vi "IV.vi"(6 "Speed":enum16{"Normal", "Fast", "Instant"}(ring), 8 "error in":errorcluster, 11 "Transport":refnum<class "SMO.Transport.lvclass">) -> (0 "error out":errorcluster, 3 "Transport out":refnum<class "SMO.Transport.lvclass">)   [LabVIEW 2019, in "SMO.Transport.lvclass"]
uses:
  SMO.Transport.lvclass
  <userlib>/LevyLab/Lockin-Multichannel/Instrument.Lockin/Instrument.Lockin.lvclass
  SMO.Control Experiment/SMO.Control Experiment.lvclass
  <userlib>/LevyLab/Instrument Framework/Instrument Types/CBridge/Instrument.CBridge.lvclass
  <userlib>/LevyLab/Instrument Framework/Instrument Types/Cryostat/Instrument.Cryostat.lvclass
  <userlib>/LevyLab/Krohn Hite 7008/Instrument.KH7008.lvclass
  <userlib>/LevyLab/Instrument Framework/Instrument Types/Strain/Instrument.Strain.lvclass
  <userlib>/LevyLab/Instrument Framework/Instrument Types/VNA/Instrument.VNA.lvclass
  <userlib>/LevyLab/Instrument Framework/Instrument Types/VSource/Instrument.VSource.lvclass
  SMO.Control Experiment/Private/Control Experiment SM/Typedefs/Instruments--cluster.ctl
  <userlib>/LevyLab/Instrument Framework/Instrument Types/Delay Line/Instrument.DelayLine.lvclass
  <userlib>/LevyLab/Lockin-Multichannel/Instrument.DAQ/Typedefs/AO.Channel.Function--Enum.ctl
  <userlib>/LevyLab/Lockin-Multichannel/Instrument.DAQ/Instrument.DAQ.lvclass
  <userlib>/LevyLab/Lockin-Multichannel/Instrument.DAQ/Typedefs/AO.Channel--Cluster.ctl
  <userlib>/LevyLab/Lockin-Multichannel/Instrument.DAQ/Typedefs/AO.Channel--Cluster--Array.ctl
  <userlib>/_OpenG.lib/array/array.llb/Index 1D Array Elements (Variant)__ogtk.vi
panel:
  out "4Term":cluster{dbl[], dbl[]}[](graph)
  out "2Term":T1(graph)
  in  "Tab Control":T2(tab)
  in  "decimating factor":i32=5
  in  "low cutoff freq: fl":dbl=0.01 format="%0.4f"
  out "Temp (K)":dbl=0.013306618000000001
  in  "offset":dbl[](array[numeric])=[0.0, 0.0, 0.0, 0.0, 0.0, 0.0, 0.0, 0.0, 0.0, 0.0, 0.0, 0.0, 0.0, 0.0, 0.0, 0.0, 0.0, 0.0, 0.0, 0.0, 0.0, 0.0, 0.0, 0.0] format="%_6p"
  in  "invert":dbl[](array[numeric])=[1.0, 1.0, 1.0, 1.0, 1.0, 1.0, 1.0, 1.0, 1.0, 1.0, 1.0, 1.0, 1.0, 1.0, 1.0, 1.0, 1.0, 1.0, 1.0, 1.0, 1.0, 1.0, 1.0, 1.0] format="%#_6p"
  out "Field (T)":dbl=-0.0014
  in  "Enable Filter?":bool
  out "AI Waveform":waveform(dbl)[](graph)
  out "AO Waveform":waveform(dbl)[](graph)
  in  "AI indices":i32[](array[numeric])
  in  "AO indices":i32[](array[numeric])
  in  "Experiment Folder":string="test"
  in  "Experiment Comments":string="   IV measurements at 0T\n     - Sweep priority 0: +y gate from 25V to -25V in steps of 2V (-y -25 to 25)\n     - 1 IV curves at each Vsg\n     - KH channel 17,18,19,20: leads 3,8,15,27\n    Vbg = lead 26: 0V\n    T: 20mK\n    B=0T\n    \n    \n    400nm periodicity mesh\n    \n        KH channel 4,3: leads 7,6 , current mode, 5k resistor, 1000x gain\n        lead 7: 5mV ac+ 0uV dc bias, 0.02 Hz\n        KH channel 1,2: V1+/-: 4,5 1000x gain\n    \n    rectangle\n    \n        KH channel 7,6: leads 12,11, current mode, 5k resistor, 1000x gain\n        lead 12: 5mV ac+ 0uV dc bias, 0.02 Hz\n        KH channel 8,5: V1+/-: 13,9 1000x gain\n    \n    \n    200nm periodicity mesh\n    \n        KH channel 12,11: leads 16,17 , current mode, 5k resistor, 1000x gain\n        lead 21: 5mV ac+ 180uV dc bias, 0.02 Hz\n        KH channel 9,10: V1+/-: 21,20 1000x gain\n    \n    line filter on in lockin\n    decimating factor: 5"
  in  "OK":bool
  # "Speed:\n- Normal: The Lockin is \"paused\" and this program triggers an aquisition and waits for a new waveform. There is some program overhead so it takes slightly longer than acquisition time\n- Fast: Set the Lockin to be in running mode with whatever acquisition time you want (1 s, 2 s, 5 s, etc) and then this program acquires the waveforms and saves them. \n- Instant: There are NO checks to make sure that the waveform is different than the previous."
  # "*** These controls are only read if this VI is the top level. If is is called from Sweep Control then the folder and comments come from Sweep Control.vi ***"
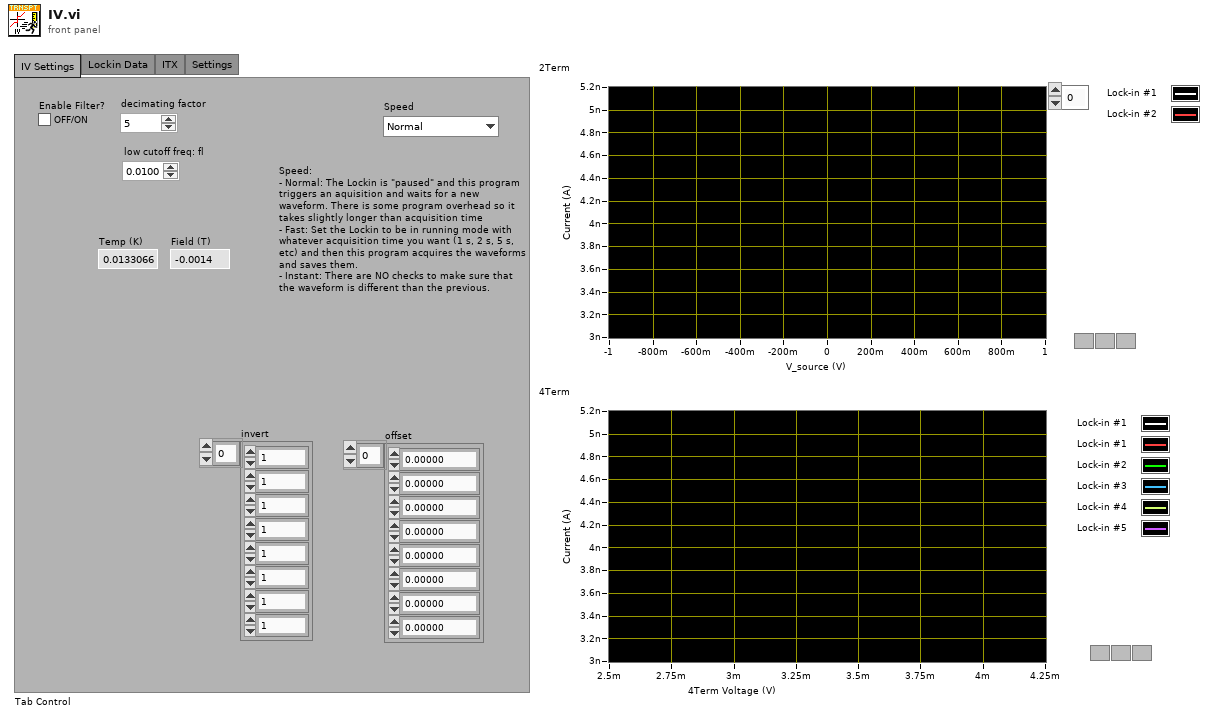
[diagram p1: front panel]
types:
  T1 = cluster{"Decimated and Filtered Array":dbl[], "Decimated and Filtered Array":dbl[]}[]
  T2 = enum32{"IV Settings", "Lockin Data", "ITX", "Settings"}
  T3 = enum32{"Invalid", "Standard", "Closed", "Hidden", "Minimized", "Maximized"}
  T4 = enum32{"invalid app kind", "Development System", "Run Time System", "Student Edition", "Embedded LabVIEW", "Evaluation", "Custom"}
  T5 = typedef "SMO.Control Experiment.lvclass/Instruments--cluster.ctl" = cluster{"Lockin":refnum<class "Instrument.Lockin.lvclass">, "Temperature":refnum<class "Instrument.Cryostat.lvclass">, "Magnet":refnum<class "Instrument.Cryostat.lvclass">, "Rotator":refnum<class "Instrument.Cryostat.lvclass">, "Level":refnum<class "Instrument.Cryostat.lvclass">, "C Bridge":refnum<class "Instrument.CBridge.lvclass">, "Optical Delay Line":refnum<class "Instrument.DelayLine.lvclass">, "Strain Cell":refnum<class "Instrument.Strain.lvclass">, "VNA":refnum<class "Instrument.VNA.lvclass">, "Voltage Source":refnum<class "Instrument.VSource.lvclass">, "KH7008":refnum<class "Instrument.KH7008.lvclass">[]}
  T6 = typedef "Instrument.DAQ.lvclass/AO.Channel--Cluster--Array.ctl" = T7[]
  T7 = typedef "Instrument.DAQ.lvclass/AO.Channel--Cluster.ctl" = cluster{"Enable?":bool, "Channel":i32, "Amplitude":dbl, "Offset":dbl, "Frequency":dbl, "Phase":dbl, "Function":T8, "Sweeping?":bool}
  T8 = typedef "Instrument.DAQ.lvclass/AO.Channel.Function--Enum.ctl" = enum16{"Sine", "Triangle", "Square"}
  T9 = cluster{"Core":cluster{"Current VI Reference":refnum<vi>, "Close Panel on Exit?":bool}, "Transport":refnum<class "SMO.Transport.lvclass">, "Control Experiment":refnum<class "SMO.Control Experiment.lvclass">, "Instruments":T5, "Temperature":dbl, "Magnet":dbl, "AOconfig":T6, "AO Waveforrm":waveform(dbl)[], "AI Waveform":waveform(dbl)[], "time":dbl[], "time (filtered)":dbl[], "AI (filtered)":cluster{"Decimated and Filtered Array":dbl[]}[], "AO (filtered)":cluster{"Decimated and Filtered Array":dbl[]}[], "Execution:State":enum32{"Bad", "Idle", "Run top level", "Running"}}
  T10 = enum32{"Bad", "Idle", "Run top level", "Running"}
  T11 = cluster{"Current VI Reference":refnum<vi>, "Close Panel on Exit?":bool}
  T12 = cluster{"I-":i32, "I+":i32, "V1-":i32, "V1+":i32, "I2-":i32, "I2+":i32, "V2-":i32, "V2+":i32}
  T13 = cluster{"Decimated and Filtered Array":dbl[], "Decimated and Filtered Array":dbl[]}
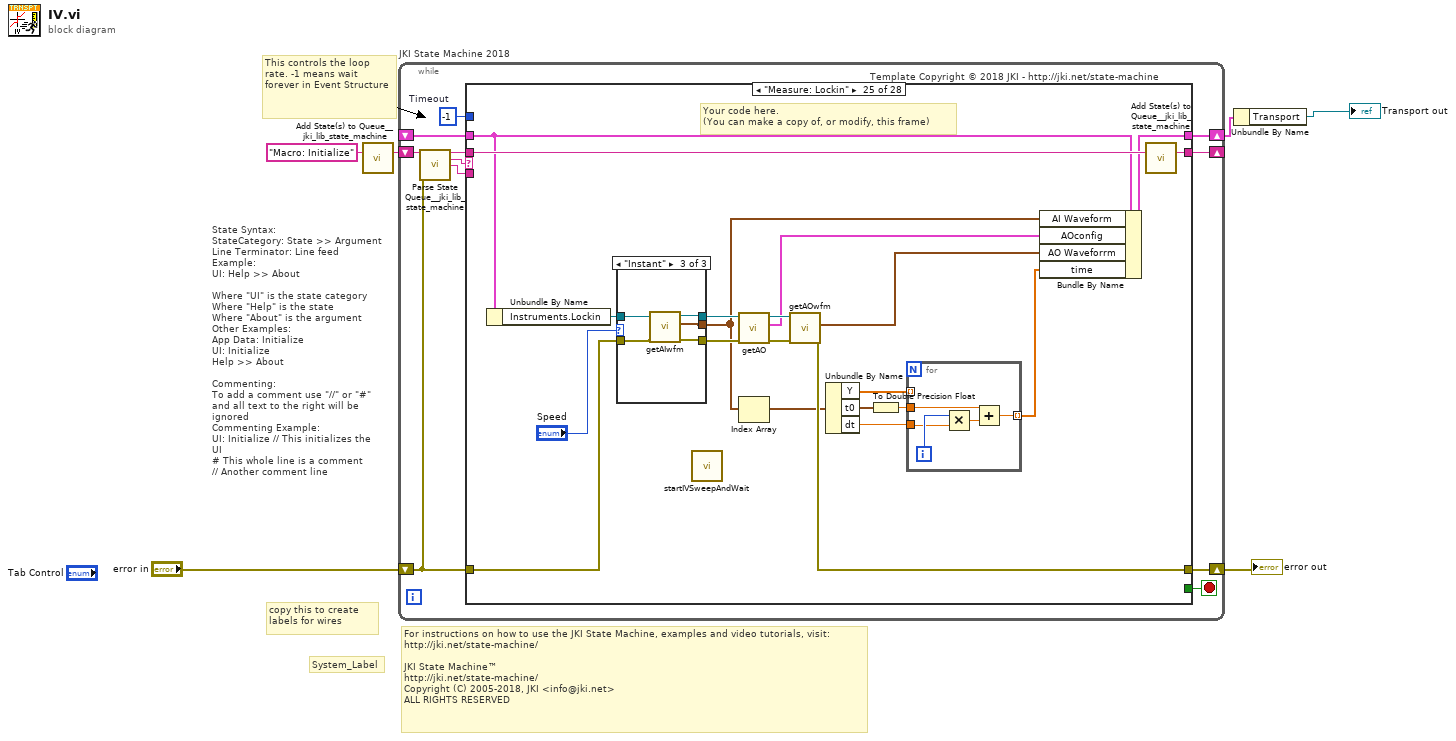
[diagram p0: block diagram]
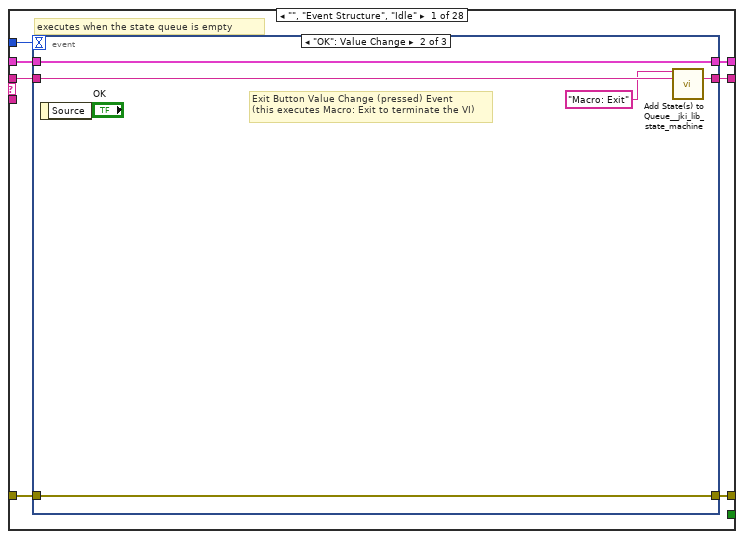
[diagram p2: hidden frame]
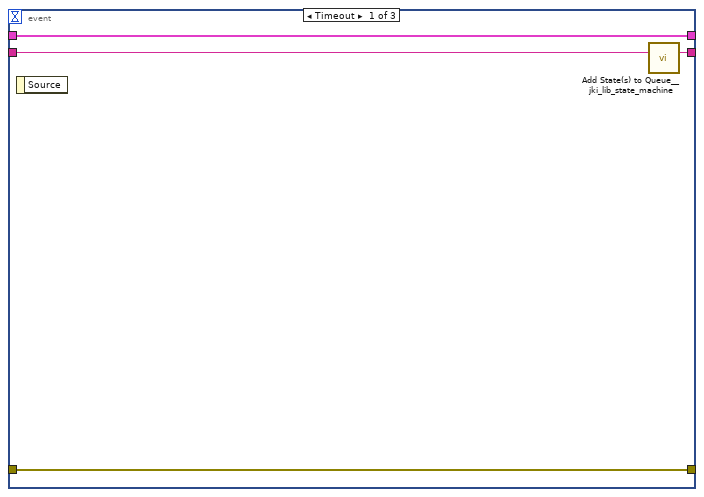
[diagram p3: hidden frame]
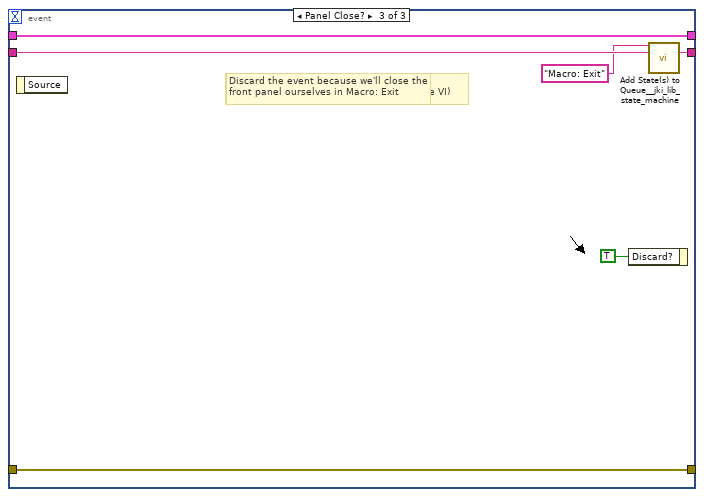
[diagram p4: hidden frame]
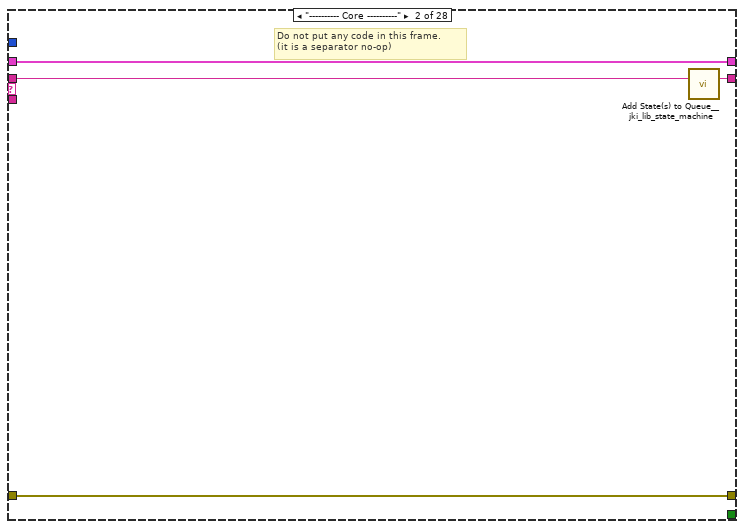
[diagram p5: hidden frame]
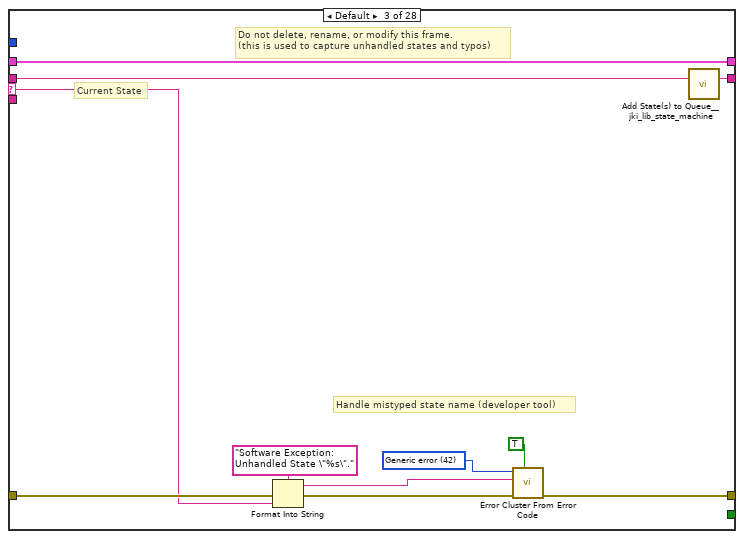
[diagram p6: hidden frame]
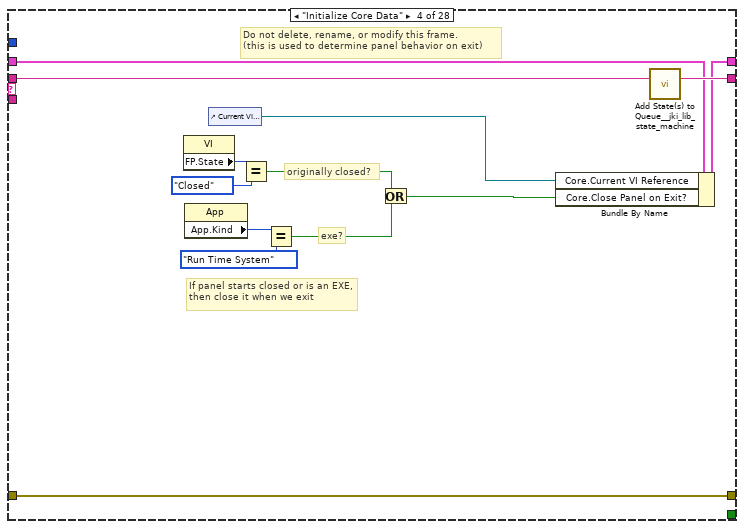
[diagram p7: hidden frame]
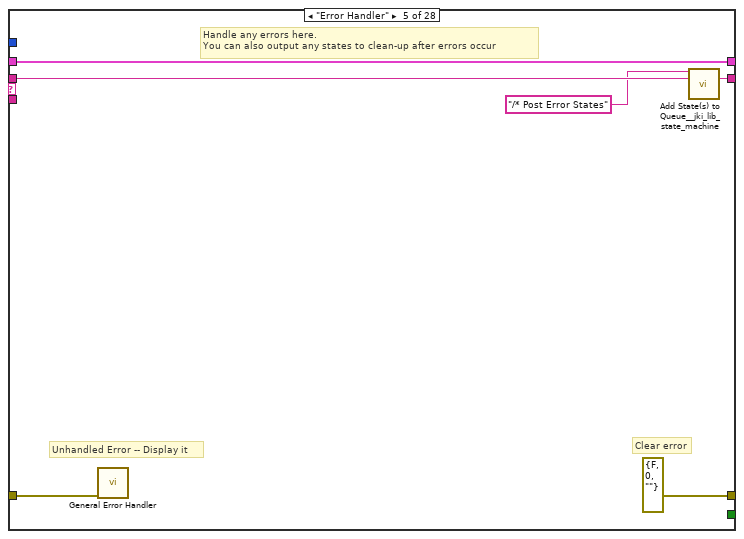
[diagram p8: hidden frame]
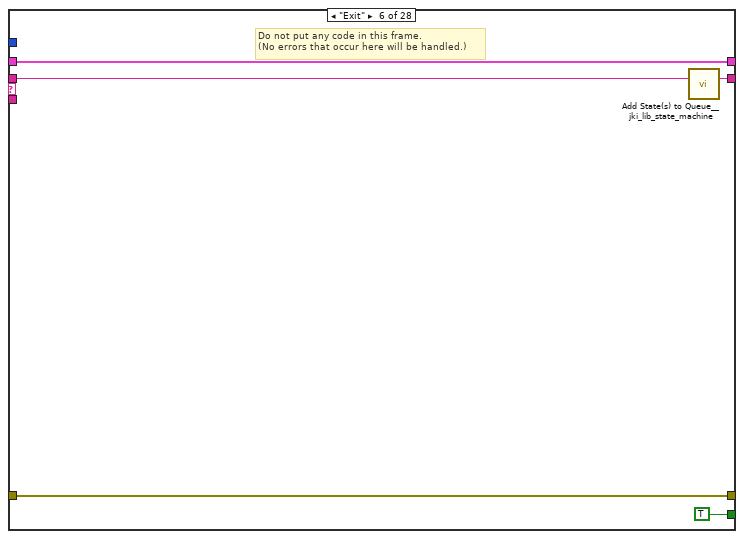
[diagram p9: hidden frame]
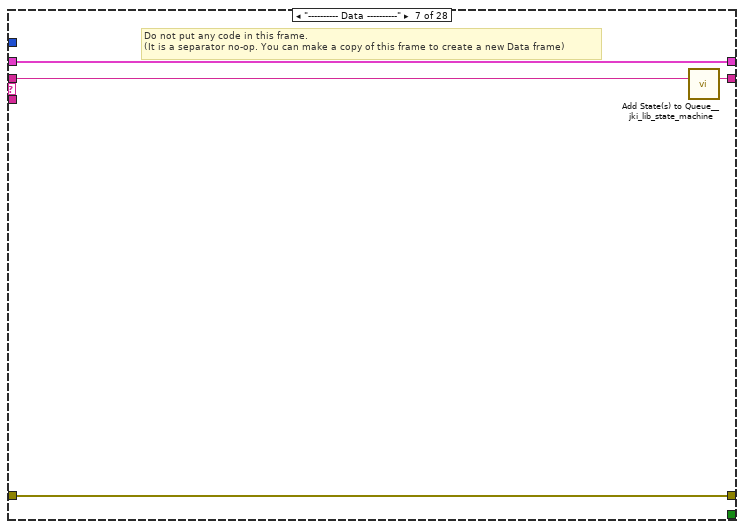
[diagram p10: hidden frame]
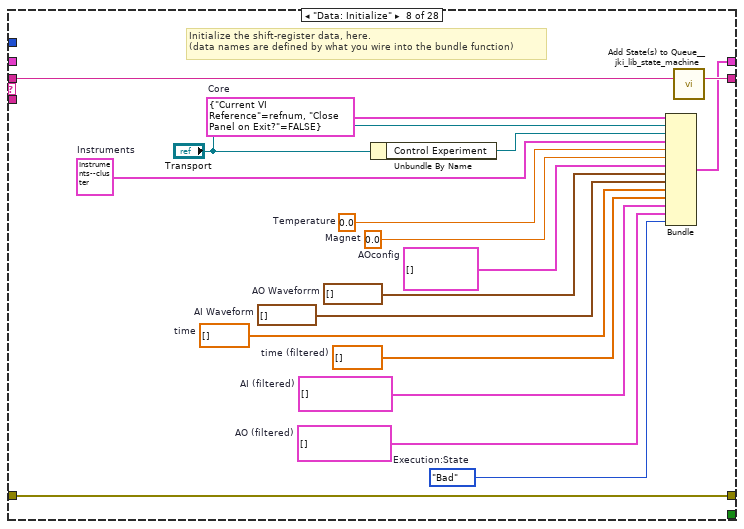
[diagram p11: hidden frame]
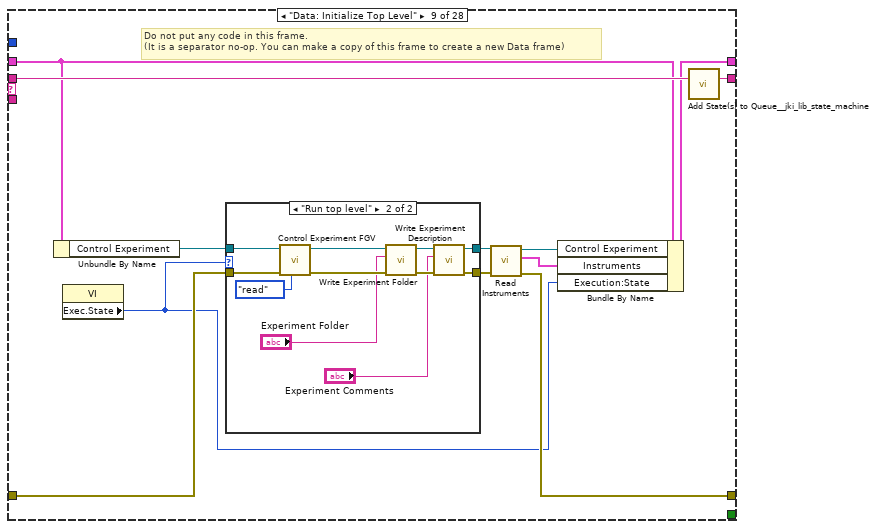
[diagram p12: hidden frame]
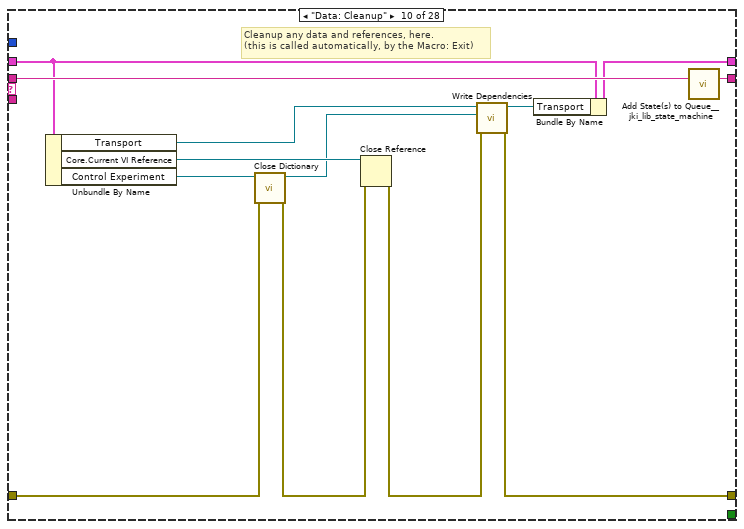
[diagram p14: hidden frame]
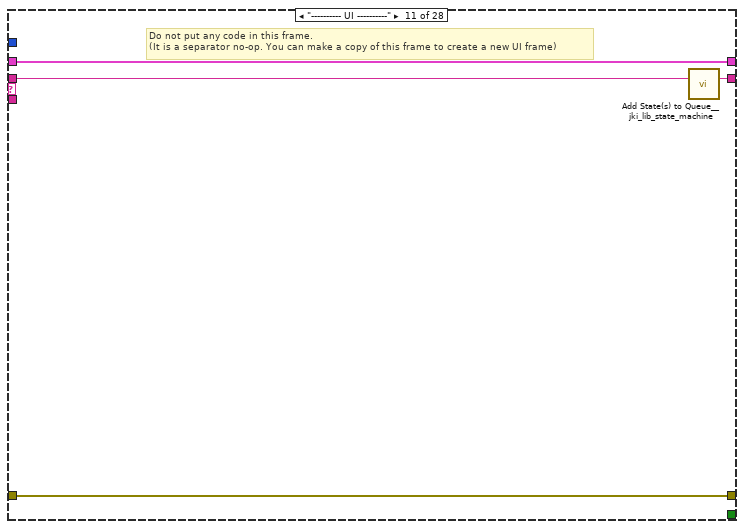
[diagram p15: hidden frame]
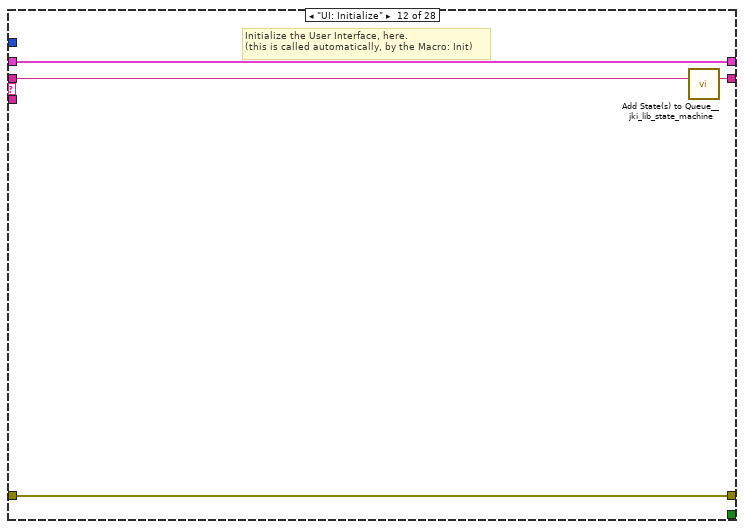
[diagram p16: hidden frame]
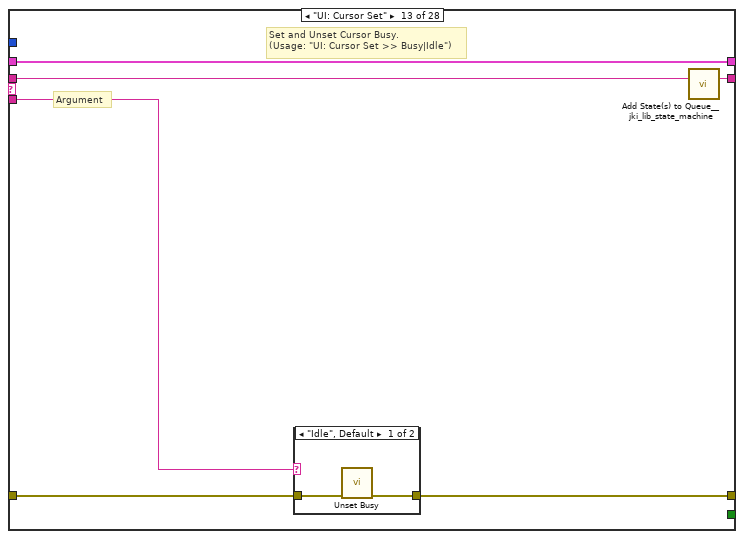
[diagram p17: hidden frame]
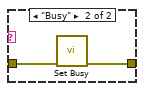
[diagram p18: hidden frame]
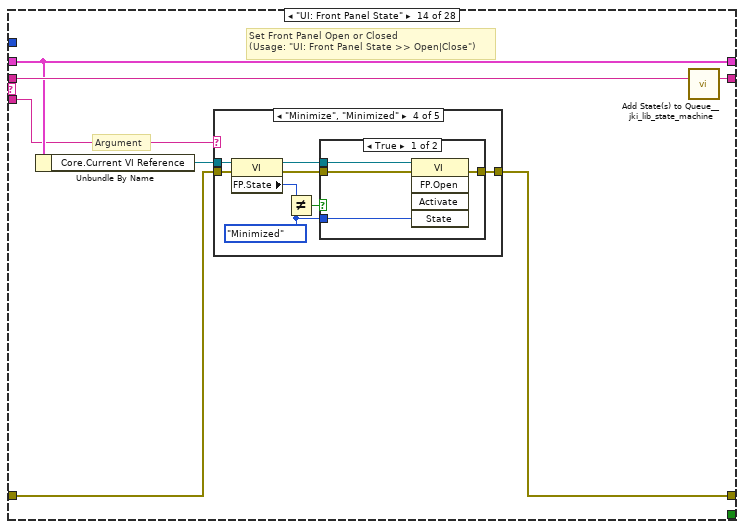
[diagram p19: hidden frame]
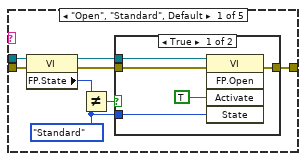
[diagram p20: hidden frame]
diagram:
  # "For instructions on how to use the JKI State Machine, examples and video tutorials, visit:\nhttp://jki.net/state-machine/\n\nJKI State Machine™\nhttp://jki.net/state-machine/\nCopyright (C) 2005-2018, JKI <info@jki.net>\nALL RIGHTS RESERVED"
  # "State Syntax:\nStateCategory: State >> Argument\nLine Terminator: Line feed\nExample:\nUI: Help >> About\n\nWhere \"UI\" is the state category\nWhere \"Help\" is the state\nWhere \"About\" is the argument\nOther Examples:\nApp Data: Initialize\nUI: Initialize\nHelp >> About\n\nCommenting:\nTo add a comment use \"//\" or \"#\" and all text to the right will be ignored\nCommenting Example:\nUI: Initialize // This initializes the UI\n# This whole line is a comment\n// Another comment line"
  # "copy this to create labels for wires"
  # "This controls the loop rate. -1 means wait forever in Event Structure"
  # "System_Label"
  n1 = call <vilib>:"Add State(s) to Queue__jki_lib_state_machine.vi"("State(s) in (\"\")"="Macro: Initialize") -> ("States Out"=w6:string)  [unwired: 14 in]
  n2 = while "JKI State Machine 2018" {
    shift-right: [w10] -> w4
    shift-left: _ -> [w9]
    shift-right: [w13] -> w1
    shift-left: "error in" -> [w7]
    shift-right: [w12] -> _
    shift-left: w6 -> [w14]
    stop <- w11 stop-if-true
    w8 = -1  # Timeout
    # "Template Copyright © 2018 JKI - http://jki.net/state-machine"
    n3 = call <vilib>:"Parse State Queue__jki_lib_state_machine.vi"("State Queue"=w14, "Error In (no error)"=w7) -> ("Remaining States"=w16:string, "Current State"=w17:string, "Arguments"=w15:string)  [unwired: 11 in]
    n4 = case shown="\"Measure: Lockin\"" w17 {
      selector: w17 -> [_ _ w44 _ _ _ _ _ _ _ _ _ _ _ _ _ _ _ _ _ _ _ _ _ _ _ _ _]
      tunnel: w16 -> [w24 w43 w48 w67 w73 w78 w82 w100 w112 w138 w142 w146 w152 w163 w240 w271 w275 w280 w290 w294 w309 w316 w331 w345 w366 w403 w424 w447]
      tunnel: w15 -> [_ _ _ _ _ _ _ _ _ _ _ _ w147 w157 _ _ _ _ _ _ _ w313 _ _ _ _ _ _]
      tunnel: w9 -> [w22 w40 w46 w60 w70 w76 w79 _ w102 w132 w139 w144 w150 w159 w237 w251 w272 w277 w287 w291 w305 w314 w329 w334 w351 w390 w421 w438]
      tunnel: [w21 w41 w50 w64 errorcluster {"status"=FALSE, "code"=0, "source"=""} ("error out") w75 w80 w97 w105 w127 w140 w143 w148 w160 w238 w244 w273 w278 w288 w292 w303 w310 w327 w343 w359 w401 w422 w445] -> w13
      tunnel: w7 -> [w20 w41 w49 w64 w69 w75 w80 w97 w106 w134 w140 w143 w149 w161 w238 w245 w273 w278 w288 w292 w306 w311 w318 w335 w360 w401 w422 w442]
      tunnel: [w23 w42 w47 w66 w72 w77 w81 w99 w111 w137 w141 w145 w151 w162 w239 w270 w274 w279 w289 w293 w308 w315 w330 w344 w365 w402 w423 w446] -> w12
      tunnel: [_ _ _ _ _ TRUE _ _ _ _ _ _ _ _ _ _ _ _ _ _ _ _ _ _ _ _ _ _] -> w11
      tunnel: [w19 w40 w46 w65 w70 w76 w79 w98 w104 w131 w139 w144 w150 w159 w237 w251 w272 w277 w287 w291 w304 w314 w328 w333 w350 w389 w421 w437] -> w10
      tunnel: w8 -> [w18 _ _ _ _ _ _ _ _ _ _ _ _ _ _ _ _ _ _ _ _ _ _ _ _ _ _ _]
      frame "", "Event Structure", "Idle" {
        # "executes when the state queue is empty"
        n5 = event shown="[1] \"OK\": Value Change" {
          selector: _ -> [_ _ _]
          dyn-events: _ -> [_ _ _]
          timeout: w18 -> [_ _ _]
          tunnel: w24 -> [w28 w33 w39]
          tunnel: [w27 w32 w38] -> w23
          tunnel: w22 -> [w25 w30 w36]
          tunnel: [w26 w31 w37] -> w21
          tunnel: w20 -> [w26 w31 w37]
          tunnel: [w25 w30 w36] -> w19
          event Timeout {
            n6 = event-data() -> ()  [unwired: 1 in, 1 out]
            n7 = call <vilib>:"Add State(s) to Queue__jki_lib_state_machine.vi"("State(s) in (\"\")"=w28) -> ("States Out"=w27:string)  [unwired: 14 in]
          }
          event "OK": Value Change {
            # "Exit Button Value Change (pressed) Event\n(this executes Macro: Exit to terminate the VI)"
            n8 = event-data() -> ()  [unwired: 1 in, 1 out]
            n9 = call <vilib>:"Add State(s) to Queue__jki_lib_state_machine.vi"("State(s) in Front (\"\")"="Macro: Exit", "State(s) in (\"\")"=w33) -> ("States Out"=w32:string)  [unwired: 13 in]
          }
          event Panel Close? {
            # "Discard the event because we'll close the front panel ourselves in Macro: Exit"
            # "Close Panel button (pressed) Event\n(this executes Macro: Exit to terminate the VI)"
            n10 = event-data() -> ()  [unwired: 1 in, 1 out]
            n11 = event-data("Discard?"=TRUE) -> ()  [unwired: 1 in, 1 out]
            n12 = call <vilib>:"Add State(s) to Queue__jki_lib_state_machine.vi"("State(s) in Front (\"\")"="Macro: Exit", "State(s) in (\"\")"=w39) -> ("States Out"=w38:string)  [unwired: 13 in]
          }
        }
      }
      frame "---------- Core ----------" {
        # "Do not put any code in this frame.\n(it is a separator no-op)"
        n13 = call <vilib>:"Add State(s) to Queue__jki_lib_state_machine.vi"("State(s) in (\"\")"=w43) -> ("States Out"=w42:string)  [unwired: 14 in]
      }
      frame Default {
        w53 = 42 items=["No error", "Argument error", "Memory is full", "Out of zone", "End of file", "File already open", "Generic file I/O error", "File not found", "File permission error", "Disk is full", "Duplicate path", "Too many files open", "System feature not enabled", "Resource file not found", "Cannot add resource", "Resource not found", "Image not found", "Image memory error", "Pen does not exist", "Config type invalid", "Config token not found", "Config parse error", "Config memory error", "Bad external code format", "Bad external code offset", "External code not present", "Null window", "Destroy window error", "Null menu", "Print aborted", "Bad print record", "Print driver error", "Windows error during printing", "Memory error during printing", "Print dialog error", "Generic print error", "Invalid device refnum", "Device not found", "Device parameter error", "Device unit error", "Cannot open device", "Device call aborted", "Generic error", "Cancelled by user", "Object ID too low", "Object ID too high", "Object not in heap", "Unknown heap", "Unknown object (invalid DefProc)", "Unknown object (DefProc not in table)", "Message out of range", "Invalid (null) method", "Unknown message", "Manager call not supported", "Bad address", "Network operation in progress", "Network operation timed out", "Connection is busy", "Network attribute not supported", "Network error", "Address in use", "System out of memory", "Connection aborted", "Connection refused", "Not connected", "Already connected", "Connection closed", "Initialization error (interapplication manager)", "Bad occurrence", "Wait on unbound occurrence handler", "Occurrence queue overflow", "Datalog type conflict", "Unused", "Unrecognized type (interapplication manager)", "Memory corrupt", "Failed to make temporary DLL", "Old CIN version", "Drag socket not found", "Failed to load drop-object", "Failed to register OLE object", "Failed to release OLE object", "Format specifier type mismatch", "Unknown format specifier", "Too few format specifiers", "Too many format specifiers", "Scan failed", "Newer CIN version", "Error converting to variant", "Runtime menu error", "Password tampered", "Variant attribute not found", "Incompatible variant data type", "Event data is not available", "Event Store is not present", "Occurrence is not found", "Event Queue is not created", "Event info is not available", "Refnum passed is NULL", "Error retrieving Class GUID", "Error retrieving CoClass GUID", "Error retrieving TypeLib GUID.", "Bad built application magic bytes.", "Specific driver is different from the specific driver associated with the Logical Name.", "There is no session opened to the class driver.", "Max Error", "MAX - Error with config objects", "MAX - Error loading configuration", "MAX - Group not supported"]
        # "Current State"
        # "Do not delete, rename, or modify this frame.\n(this is used to capture unhandled states and typos)"
        # "Handle mistyped state name (developer tool)"
        n14 = Format Into String(format string="Software Exception: Unhandled State \"%s\"." ("message"), error in=w49, w44) -> (resulting string=w52:string, error out=w51:errorcluster)  [unwired: 1 in]
        n15 = call <vilib>:"Error Cluster From Error Code.vi"("show call chain? (False)"=TRUE, "error in (no error)"=w51, "error message (\"\")"=w52, "error code (0)"=w53) -> ("error out"=w50:errorcluster)  [unwired: 5 in]
        n16 = call <vilib>:"Add State(s) to Queue__jki_lib_state_machine.vi"("State(s) in (\"\")"=w48) -> ("States Out"=w47:string)  [unwired: 14 in]
      }
      frame "Initialize Core Data" {
        # "Do not delete, rename, or modify this frame.\n(this is used to determine panel behavior on exit)"
        # "originally closed?"
        # "exe?"
        # "If panel starts closed or is an EXE, then close it when we exit"
        n17 = property class="VI"() -> ("FP.State"=w57:T3)  [unwired: 2 in, 2 out]
        n18 = property class="App"() -> ("App.Kind"=w63:T4)  [unwired: 2 in, 2 out]
        n19 = control-ref of="Current VI Reference"() -> (w58:refnum<vi>)
        n20 = Equal?(x=w57, y=T3."Closed" ("Front Panel Window:State")) -> (x = y?=w55:bool)
        n21 = Equal?(x=w63, y=T4."Run Time System" ("Application:Kind")) -> (x = y?=w61:bool)
        n22 = Or(x=w55, y=w61) -> (x .or. y?=w59:bool)
        n23 = Bundle By Name(cluster=w60, "Core.Current VI Reference"=w58, "Core.Close Panel on Exit?"=w59) -> (w65:T9)
        n24 = call <vilib>:"Add State(s) to Queue__jki_lib_state_machine.vi"("State(s) in (\"\")"=w67) -> ("States Out"=w66:string)  [unwired: 14 in]
      }
      frame "Error Handler" {
        # "Unhandled Error -- Display it"
        # "Handle any errors here.\nYou can also output any states to clean-up after errors occur"
        # "Clear error"
        n25 = call <vilib>:"General Error Handler.vi"("error in (no error)"=w69) -> ()  [unwired: 10 in, 5 out]
        n26 = call <vilib>:"Add State(s) to Queue__jki_lib_state_machine.vi"("State(s) in Front (\"\")"="/* Post Error States", "State(s) in (\"\")"=w73) -> ("States Out"=w72:string)  [unwired: 13 in]
      }
      frame "Exit" {
        # "Do not put any code in this frame.\n(No errors that occur here will be handled.)"
        n27 = call <vilib>:"Add State(s) to Queue__jki_lib_state_machine.vi"("State(s) in (\"\")"=w78) -> ("States Out"=w77:string)  [unwired: 14 in]
      }
      frame "---------- Data ----------" {
        # "Do not put any code in this frame.\n(It is a separator no-op. You can make a copy of this frame to create a new Data frame)"
        n28 = call <vilib>:"Add State(s) to Queue__jki_lib_state_machine.vi"("State(s) in (\"\")"=w82) -> ("States Out"=w81:string)  [unwired: 14 in]
      }
      frame "Data: Initialize" {
        w84 = T5 {"Lockin"=refnum, "Temperature"=refnum, "Magnet"=refnum, "Rotator"=refnum, "Level"=refnum, "C Bridge"=refnum, "Optical Delay Line"=refnum, "Strain Cell"=refnum, "VNA"=refnum, "Voltage Source"=refnum, "KH7008"=[]}  # Instruments
        w85 = T10."Bad"  # Execution:State
        w86 = 0.0  # Magnet
        w87 = 0.0  # Temperature
        w88 = cluster{"Decimated and Filtered Array":dbl[]}[] []  # AO (filtered)
        w89 = cluster{"Decimated and Filtered Array":dbl[]}[] []  # AI (filtered)
        w90 = dbl[] []  # time (filtered)
        w91 = dbl[] []  # time
        w93 = waveform(dbl)[] []  # AO Waveforrm
        w94 = T6 []  # AOconfig
        w92 = waveform(dbl)[] []  # AI Waveform
        w96 = T11 {"Current VI Reference"=refnum, "Close Panel on Exit?"=FALSE}  # Core
        # "Initialize the shift-register data, here.\n(data names are defined by what you wire into the bundle function)"
        n29 = Unbundle By Name("Transport") -> ("Control Experiment"=w95:refnum<class "SMO.Control Experiment.lvclass">)
        n30 = Bundle("Core"=w96, "Transport"="Transport", "Control Experiment"=w95, "Instruments"=w84, "Temperature"=w87, "Magnet"=w86, "AOconfig"=w94, "AO Waveforrm"=w93, "AI Waveform"=w92, "time"=w91, "time (filtered)"=w90, "AI (filtered)"=w89, "AO (filtered)"=w88, "Execution:State"=w85) -> (w98:T9)  [unwired: 1 in]
        n31 = call <vilib>:"Add State(s) to Queue__jki_lib_state_machine.vi"("State(s) in (\"\")"=w100) -> ("States Out"=w99:string)  [unwired: 14 in]
      }
      frame "Data: Initialize Top Level" {
        # "Do not put any code in this frame.\n(It is a separator no-op. You can make a copy of this frame to create a new Data frame)"
        n32 = Unbundle By Name(w102) -> ("Control Experiment"=w103:refnum<class "SMO.Control Experiment.lvclass">)
        n33 = property class="VI"() -> ("Exec.State"=w101:T10)  [unwired: 2 in, 2 out]
        n34 = case shown="\"Run top level\"" w101 {
          tunnel: [w114 w121] -> w108
          tunnel: [w113 w120] -> w107
          tunnel: w106 -> [w114 w119]
          tunnel: w103 -> [w113 w115]
          frame "Running", Default {
          }
          frame "Run top level" {
            n35 = call "Control Experiment FGV.vi"("Function"=enum16{"read", "write"}."read", "error in (no error)"=w119, "Control Experiment"=w115) -> ("error out"=w124:errorcluster, "Control Experiment out"=w125:refnum<class "SMO.Control Experiment.lvclass">)  [unwired: 7 in]
            n36 = call "Write Experiment Folder.vi"("error in (no error)"=w124, "Experiment Folder"="Experiment Folder", "Control Experiment"=w125) -> ("error out"=w122:errorcluster, "Control Experiment out"=w123:refnum<class "SMO.Control Experiment.lvclass">)  [unwired: 7 in]
            n37 = call "Write Experiment Description.vi"("error in (no error)"=w122, "Experiment Description"="Experiment Comments", "Control Experiment"=w123) -> ("error out"=w121:errorcluster, "Control Experiment out"=w120:refnum<class "SMO.Control Experiment.lvclass">)  [unwired: 7 in]
          }
        }
        n38 = call "Read Instruments.vi"("error in (no error)"=w108, "Control Experiment"=w107) -> ("error out"=w105:errorcluster, "Instruments"=w109:T5, "Control Experiment out"=w110:refnum<class "SMO.Control Experiment.lvclass">)  [unwired: 7 in]
        n39 = Bundle By Name(cluster=w102, "Control Experiment"=w110, "Instruments"=w109, "Execution:State"=w101) -> (w104:T9)
        n40 = call <vilib>:"Add State(s) to Queue__jki_lib_state_machine.vi"("State(s) in (\"\")"=w112) -> ("States Out"=w111:string)  [unwired: 14 in]
      }
      frame "Data: Cleanup" {
        # "Cleanup any data and references, here.\n(this is called automatically, by the Macro: Exit)"
        n41 = Unbundle By Name(w132) -> ("Transport"=w129:refnum<class "SMO.Transport.lvclass">, "Core.Current VI Reference"=w136:refnum<vi>, "Control Experiment"=w135:refnum<class "SMO.Control Experiment.lvclass">)
        n42 = call "Close Dictionary.vi"("error in (no error)"=w134, "Control Experiment"=w135) -> ("error out"=w133:errorcluster, "Control Experiment out"=w126:refnum<class "SMO.Control Experiment.lvclass">)  [unwired: 8 in]
        n43 = Close Reference(reference=w136, error in (no error)=w133) -> (error out=w128:errorcluster)
        n44 = call "Write Dependencies.vi"("error in (no error)"=w128, "Control Experiment"=w126, "Transport in"=w129) -> ("error out"=w127:errorcluster, "Transport out"=w130:refnum<class "SMO.Transport.lvclass">)  [unwired: 7 in]
        n45 = Bundle By Name(cluster=w132, "Transport"=w130) -> (w131:T9)
        n46 = call <vilib>:"Add State(s) to Queue__jki_lib_state_machine.vi"("State(s) in (\"\")"=w138) -> ("States Out"=w137:string)  [unwired: 14 in]
      }
      frame "---------- UI ----------" {
        # "Do not put any code in this frame.\n(It is a separator no-op. You can make a copy of this frame to create a new UI frame)"
        n47 = call <vilib>:"Add State(s) to Queue__jki_lib_state_machine.vi"("State(s) in (\"\")"=w142) -> ("States Out"=w141:string)  [unwired: 14 in]
      }
      frame "UI: Initialize" {
        # "Initialize the User Interface, here.\n(this is called automatically, by the Macro: Init)"
        n48 = call <vilib>:"Add State(s) to Queue__jki_lib_state_machine.vi"("State(s) in (\"\")"=w146) -> ("States Out"=w145:string)  [unwired: 14 in]
      }
      frame "UI: Cursor Set" {
        # "Argument"
        # "Set and Unset Cursor Busy.\n(Usage: \"UI: Cursor Set >> Busy|Idle\")"
        n49 = case shown="\"Idle\", Default" w147 {
          tunnel: w149 -> [w154 w156]
          tunnel: [w153 w155] -> w148
          frame "Idle", Default {
            n50 = call <vilib>:"Unset Busy.vi"("error in (no error)"=w154) -> ("error out"=w153:errorcluster)  [unwired: 10 in]
          }
          frame "Busy" {
            n51 = call <vilib>:"Set Busy.vi"("error in (no error)"=w156) -> ("error out"=w155:errorcluster)  [unwired: 9 in, 1 out]
          }
        }
        n52 = call <vilib>:"Add State(s) to Queue__jki_lib_state_machine.vi"("State(s) in (\"\")"=w152) -> ("States Out"=w151:string)  [unwired: 14 in]
      }
      frame "UI: Front Panel State" {
        # "Argument"
        # "Set Front Panel Open or Closed\n(Usage: \"UI: Front Panel State >> Open|Close\")"
        n53 = Unbundle By Name(w159) -> ("Core.Current VI Reference"=w158:refnum<vi>)
        n54 = case shown="\"Minimize\", \"Minimized\"" w157 {
          tunnel: w161 -> [w169 w184 w195 w208 w221]
          tunnel: [w171 w185 w197 w210 w223] -> w160
          tunnel: w158 -> [w170 w182 w196 w209 w222]
          frame "Open", "Standard", Default {
            w164 = T3."Standard" ("State")
            n55 = property class="VI"(reference=w170, error in=w169) -> (reference out=w167:refnum<vi>, error out=w168:errorcluster, "FP.State"=w166:T3)
            n56 = Not Equal?(x=w166, y=w164) -> (x != y?=w165:bool)
            n57 = case shown="True" w165 {
              tunnel: [w175 w177] -> w171
              tunnel: w168 -> [w174 w177]
              tunnel: w167 -> [w173 _]
              tunnel: w164 -> [w172 _]
              frame True {
                n58 = invoke class="VI" method="FP.Open"(reference=w173, error in=w174, "Activate"=TRUE, "State"=w172) -> (error out=w175:errorcluster)  [unwired: 1 in, 4 out]
              }
              frame False {
              }
            }
          }
          frame "Close", "Closed" {
            n59 = property class="VI"(reference=w182, error in=w184) -> (reference out=w181:refnum<vi>, error out=w183:errorcluster, "FP.State"=w179:T3)
            n60 = Not Equal?(x=w179, y=T3."Closed" ("Front Panel Window:State")) -> (x != y?=w178:bool)
            n61 = case shown="True" w178 {
              tunnel: [w186 w189] -> w185
              tunnel: w183 -> [w186 w188]
              tunnel: w181 -> [_ w187]
              frame False {
              }
              frame True {
                n62 = invoke class="VI" method="FP.Close"(reference=w187, error in=w188) -> (error out=w189:errorcluster)  [unwired: 1 in, 2 out]
              }
            }
          }
          frame "Hidden", "Hide" {
            w190 = T3."Hidden" ("State")
            n63 = property class="VI"(reference=w196, error in=w195) -> (reference out=w193:refnum<vi>, error out=w194:errorcluster, "FP.State"=w192:T3)
            n64 = Not Equal?(x=w192, y=w190) -> (x != y?=w191:bool)
            n65 = case shown="True" w191 {
              tunnel: [w201 w202] -> w197
              tunnel: w194 -> [w200 w202]
              tunnel: w193 -> [w199 _]
              tunnel: w190 -> [w198 _]
              frame True {
                n66 = invoke class="VI" method="FP.Open"(reference=w199, error in=w200, "State"=w198) -> (error out=w201:errorcluster)  [unwired: 2 in, 4 out]
              }
              frame False {
              }
            }
          }
          frame "Minimize", "Minimized" {
            w203 = T3."Minimized" ("State")
            n67 = property class="VI"(reference=w209, error in=w208) -> (reference out=w206:refnum<vi>, error out=w207:errorcluster, "FP.State"=w205:T3)
            n68 = Not Equal?(x=w205, y=w203) -> (x != y?=w204:bool)
            n69 = case shown="True" w204 {
              tunnel: [w214 w215] -> w210
              tunnel: w207 -> [w213 w215]
              tunnel: w206 -> [w212 _]
              tunnel: w203 -> [w211 _]
              frame True {
                n70 = invoke class="VI" method="FP.Open"(reference=w212, error in=w213, "State"=w211) -> (error out=w214:errorcluster)  [unwired: 2 in, 4 out]
              }
              frame False {
              }
            }
          }
          frame "Maximize", "Maximized" {
            w216 = T3."Maximized" ("State")
            n71 = property class="VI"(reference=w222, error in=w221) -> (reference out=w219:refnum<vi>, error out=w220:errorcluster, "FP.State"=w218:T3)
            n72 = Not Equal?(x=w218, y=w216) -> (x != y?=w217:bool)
            n73 = case shown="True" w217 {
              tunnel: [w227 w228] -> w223
              tunnel: w220 -> [w226 w228]
              tunnel: w219 -> [w225 _]
              tunnel: w216 -> [w224 _]
              frame True {
                n74 = invoke class="VI" method="FP.Open"(reference=w225, error in=w226, "State"=w224) -> (error out=w227:errorcluster)  [unwired: 2 in, 4 out]
              }
              frame False {
              }
            }
          }
        }
        n75 = call <vilib>:"Add State(s) to Queue__jki_lib_state_machine.vi"("State(s) in (\"\")"=w163) -> ("States Out"=w162:string)  [unwired: 14 in]
      }
      frame "UI: Update Input Graphs" {
        # "Do not put any code in this frame.\n(It is a separator no-op. You can make a copy of this frame to create a new UI frame)"
        n76 = Unbundle By Name(w237) -> ("AO Waveforrm"=w230:waveform(dbl)[], "AI Waveform"=w235:waveform(dbl)[])
        n77 = call-poly <userlib>:"Index Array Elements__ogtk.vi"("indices"="AO indices", "array"=w230) -> ("elements"=w232:variant[])  [unwired: 9 in]
        n78 = Variant To Data(type=w230, Variant=w232) -> (data=→"AO Waveform":waveform(dbl)[])  [unwired: 1 in, 1 out]
        n79 = call-poly <userlib>:"Index Array Elements__ogtk.vi"("indices"="AI indices", "array"=w235) -> ("elements"=w236:variant[])  [unwired: 9 in]
        n80 = Variant To Data(type=w235, Variant=w236) -> (data=→"AI Waveform":waveform(dbl)[])  [unwired: 1 in, 1 out]
        n81 = call <vilib>:"Add State(s) to Queue__jki_lib_state_machine.vi"("State(s) in (\"\")"=w240) -> ("States Out"=w239:string)  [unwired: 14 in]
      }
      frame "UI: Update IV Graphs" {
        # "Decimated AO"
        # "Decimataed AI"
        # "Do not put any code in this frame.\n(It is a separator no-op. You can make a copy of this frame to create a new UI frame)"
        n82 = Unbundle By Name(w251) -> ("AI (filtered)"=w250:cluster{"Decimated and Filtered Array":dbl[]}[], "AO (filtered)"=w249:cluster{"Decimated and Filtered Array":dbl[]}[], "Control Experiment"=w246:refnum<class "SMO.Control Experiment.lvclass">)
        n83 = call "Get Channel Indices.vi"("error in (no error)"=w245, "Control Experiment"=w246) -> ("error out"=w244:errorcluster, "Indices"=w241:T12)  [unwired: 7 in, 1 out]
        n84 = Unbundle By Name(w241) -> ("I-"=w248:i32, "V1+"=w242:i32, "V1-"=w243:i32, "I+"=w247:i32)
        n85 = Decrement(x=w248) -> (x-1=w254:i32)
        n86 = Decrement(x=w242) -> (x-1=w263:i32)
        n87 = Decrement(x=w243) -> (x-1=w257:i32)
        n88 = Decrement(x=w247) -> (x-1=w266:i32)
        n89 = Index Array(array=w249, index=w266) -> (element=w267:cluster{"Decimated and Filtered Array":dbl[]})
        n90 = Index Array(array=w250, index #1=w254, index #2=w263, index #3=w257) -> (element #1=w260:cluster{"Decimated and Filtered Array":dbl[]}, element #2=w256:cluster{"Decimated and Filtered Array":dbl[]}, element #3=w262:cluster{"Decimated and Filtered Array":dbl[]})
        n91 = Equal?(x=w263, y=w257) -> (x = y?=w258:bool)
        n92 = Subtract(x=w256, y=w262) -> (x-y=w255:cluster{"Decimated and Filtered Array":dbl[]})
        n93 = Select(t=w256, s=w258, f=w255) -> (s? t:f=w259:cluster{"Decimated and Filtered Array":dbl[]})
        n94 = Unbundle(w260) -> ("Decimated and Filtered Array"=w264:dbl[])
        n95 = Unbundle(w267) -> ("Decimated and Filtered Array"=w265:dbl[])
        n96 = Unbundle(w259) -> ("Decimated and Filtered Array"=w261:dbl[])
        n97 = Bundle("Decimated and Filtered Array"=w261, "Decimated and Filtered Array"=w264) -> (w252:T13)  [unwired: 1 in]
        n98 = Bundle("Decimated and Filtered Array"=w265, "Decimated and Filtered Array"=w264) -> (w268:T13)  [unwired: 1 in]
        n99 = Build Array(w252) -> (→"4Term":T1)
        n100 = Build Array(w268) -> (→"2Term":T1)
        n101 = call <vilib>:"Add State(s) to Queue__jki_lib_state_machine.vi"("State(s) in (\"\")"=w271) -> ("States Out"=w270:string)  [unwired: 14 in]
      }
      frame "---------- Macro ----------" {
        # "Do not put any code in this frame.\n(It is a separator no-op. You can make a copy of this frame to create a new Macro frame)"
        n102 = call <vilib>:"Add State(s) to Queue__jki_lib_state_machine.vi"("State(s) in (\"\")"=w275) -> ("States Out"=w274:string)  [unwired: 14 in]
      }
      frame "Macro: Initialize" {
        # "Initialization Macro\n(This is called once, when the VI starts)"
        n103 = call <vilib>:"Add State(s) to Queue__jki_lib_state_machine.vi"("State(s) in Front (\"\")"="Data: Initialize\nInitialize Core Data\nUI: Initialize\nUI: Front Panel State >> Open\nData: Initialize Top Level\nMeasure: Temperature\nMeasure: Magnet\nMeasure: Capacitance\nMeasure: Wait >> 000\nMeasure: Lockin\nMeasure: Filter and Decimate\nUI: Update Input Graphs\nUI: Update IV Graphs\nFile: Save\nMacro: Exit", "State(s) in (\"\")"=w280) -> ("States Out"=w279:string)  [unwired: 13 in]
      }
      frame "Macro: Exit" {
        # "Exit Macro\n(This is called once, when the VI exits)"
        n104 = Unbundle By Name(w287) -> ("Core.Close Panel on Exit?"=w286:bool)
        n105 = Select(t="UI: Front Panel State >> Close", s=w286, f="") -> (s? t:f=w283:string)
        n106 = call <vilib>:"Add State(s) to Queue__jki_lib_state_machine.vi"("State(s) in (\"\")"=w283, "State(s) at Back (\"\")"="Data: Cleanup\nExit") -> ("States Out"=w281:string)  [unwired: 13 in]
        n107 = call <vilib>:"Add State(s) to Queue__jki_lib_state_machine.vi"("State(s) in Front (\"\")"=w281, "State(s) in (\"\")"=w290) -> ("States Out"=w289:string)  [unwired: 13 in]
      }
      frame "---------- Measure ----------" {
        # "Template Separator\n(You can make a copy of, or modify, this frame)"
        n108 = call <vilib>:"Add State(s) to Queue__jki_lib_state_machine.vi"("State(s) in (\"\")"=w294) -> ("States Out"=w293:string)  [unwired: 14 in]
      }
      frame "Measure: Temperature" {
        # "Your code here.\n(You can make a copy of, or modify, this frame)"
        n109 = Unbundle By Name(w305) -> ("Control Experiment"=w299:refnum<class "SMO.Control Experiment.lvclass">, "Instruments.Temperature"=w307:refnum<class "Instrument.Cryostat.lvclass">)
        n110 = call-dynamic "Get Temperature.vi"("error in (no error)"=w306, "Instrument.Cryostat in"=w307) -> ("error out"=w300:errorcluster, "Temperature (K)"=w296:dbl, "Instrument.Cryostat out"=w295:refnum<class "Instrument.Cryostat.lvclass">)  [unwired: 5 in, 2 out]
        "Temp (K)" <- w296
        n111 = call "Write Dictionary Element.vi"("error in (no error)"=w300, "value"=w296, "key"="Temperature", "Control Experiment"=w299) -> ("error out"=w298:errorcluster, "Control Experiment out"=w297:refnum<class "SMO.Control Experiment.lvclass">)  [unwired: 6 in]
        n112 = Bundle By Name(cluster=w305, "Instruments.Temperature"=w295, "Control Experiment"=w297) -> (w304:T9)
        n113 = call <vilib>:"Clear Errors.vi"("error in (no error)"=w298, "specific error code to clear (0: all)"=4000) -> ("error out"=w303:errorcluster)  [unwired: 4 in, 1 out]
        n114 = call <vilib>:"Add State(s) to Queue__jki_lib_state_machine.vi"("State(s) in (\"\")"=w309) -> ("States Out"=w308:string)  [unwired: 14 in]
      }
      frame "Measure: Wait" {
        # "Template Separator\n(You can make a copy of, or modify, this frame)"
        n115 = Scan From String(input string=w313) -> (output 1=w312:dbl)  [unwired: 4 in, 3 out]
        n116 = call <userlib>:"Wait (ms)__ogtk.vi"("error in (no error)"=w311, "milliseconds to wait"=w312) -> ("error out"=w310:errorcluster)  [unwired: 8 in, 1 out]
        n117 = call <vilib>:"Add State(s) to Queue__jki_lib_state_machine.vi"("State(s) in (\"\")"=w316) -> ("States Out"=w315:string)  [unwired: 14 in]
      }
      frame "Measure: Magnet" {
        # "Your code here.\n(You can make a copy of, or modify, this frame)"
        n118 = Unbundle By Name(w329) -> ("Control Experiment"=w325:refnum<class "SMO.Control Experiment.lvclass">, "Instruments.Magnet"=w322:refnum<class "Instrument.Cryostat.lvclass">)
        n119 = call-dynamic "Get Magnet.vi"("error in (no error)"=w318, "Instrument.Cryostat in"=w322) -> ("error out"=w321:errorcluster, "B Field (T)"=w320:dbl, "Instrument.Cryostat out"=w317:refnum<class "Instrument.Cryostat.lvclass">)  [unwired: 5 in, 2 out]
        "Field (T)" <- w320
        n120 = call "Write Dictionary Element.vi"("error in (no error)"=w321, "value"=w320, "key"="Magnet", "Control Experiment"=w325) -> ("error out"=w323:errorcluster, "Control Experiment out"=w319:refnum<class "SMO.Control Experiment.lvclass">)  [unwired: 6 in]
        n121 = Bundle By Name(cluster=w329, "Instruments.Magnet"=w317, "Control Experiment"=w319) -> (w328:T9)
        n122 = call <vilib>:"Clear Errors.vi"("error in (no error)"=w323, "specific error code to clear (0: all)"=4000) -> ("error out"=w327:errorcluster)  [unwired: 4 in, 1 out]
        n123 = call <vilib>:"Add State(s) to Queue__jki_lib_state_machine.vi"("State(s) in (\"\")"=w331) -> ("States Out"=w330:string)  [unwired: 14 in]
      }
      frame "Measure: Capacitance" {
        # "Your code here.\n(You can make a copy of, or modify, this frame)"
        n124 = Unbundle By Name(w334) -> ("Control Experiment"=w341:refnum<class "SMO.Control Experiment.lvclass">, "Instruments.C Bridge"=w338:refnum<class "Instrument.CBridge.lvclass">)
        n125 = call-dynamic "Get Capacitance.vi"("error in (no error)"=w335, "Instrument.CBridge in"=w338) -> ("error out"=w337:errorcluster, "Capacitance (pF)"=w336:dbl)  [unwired: 7 in, 1 out]
        n126 = call "Write Dictionary Element.vi"("error in (no error)"=w337, "value"=w336, "key"="Capacitance", "Control Experiment"=w341) -> ("error out"=w339:errorcluster, "Control Experiment out"=w332:refnum<class "SMO.Control Experiment.lvclass">)  [unwired: 6 in]
        n127 = Bundle By Name(cluster=w334, "Control Experiment"=w332) -> (w333:T9)
        n128 = call <vilib>:"Clear Errors.vi"("error in (no error)"=w339, "specific error code to clear (0: all)"=4000) -> ("error out"=w343:errorcluster)  [unwired: 4 in, 1 out]
        n129 = call <vilib>:"Add State(s) to Queue__jki_lib_state_machine.vi"("State(s) in (\"\")"=w345) -> ("States Out"=w344:string)  [unwired: 14 in]
      }
      frame "Measure: Lockin" {
        # "Your code here.\n(You can make a copy of, or modify, this frame)"
        n130 = Unbundle By Name(w351) -> ("Instruments.Lockin"=w358:refnum<class "Instrument.Lockin.lvclass">)
        n131 = case shown="\"Instant\"" "Speed" {
          tunnel: [w371 w374 w377] -> w363
          tunnel: [w370 w373 w379] -> w362
          tunnel: w360 -> [w369 w376 w380]
          tunnel: w358 -> [w368 w375 w381]
          tunnel: [w367 w372 w378] -> w349
          frame "Normal", Default {
            n132 = call <userlib>:"startIVAndWait.vi"("error in (no error)"=w369, "Instrument.Lockin in"=w368) -> ("error out"=w370:errorcluster, "AI Waveform"=w367:waveform(dbl)[], "Instrument.Lockin out"=w371:refnum<class "Instrument.Lockin.lvclass">)  [unwired: 7 in]
          }
          frame "Fast" {
            n133 = call <userlib>:"waitForNewWaveforms.vi"("error in (no error)"=w376, "Instrument.Lockin in"=w375) -> ("error out"=w373:errorcluster, "Newest AI Waveform"=w372:waveform(dbl)[], "Instrument.Lockin out"=w374:refnum<class "Instrument.Lockin.lvclass">)  [unwired: 7 in]
          }
          frame "Instant" {
            n134 = call <userlib>:"getAIwfm.vi"("error in (no error)"=w380, "Instrument.Lockin in"=w381) -> ("error out"=w379:errorcluster, "AI Waveform"=w378:waveform(dbl)[], "Instrument.Lockin out"=w377:refnum<class "Instrument.Lockin.lvclass">)  [unwired: 7 in]
          }
        }
        n135 = call <userlib>:"startIVSweepAndWait.vi"() -> ()  [unwired: 10 in, 2 out]
        n136 = call <userlib>:"getAO.vi"("error in (no error)"=w362, "Instrument.Lockin in"=w363) -> ("error out"=w361:errorcluster, "AOconfig"=w357:T6, "Instrument.Lockin out"=w364:refnum<class "Instrument.Lockin.lvclass">)  [unwired: 7 in]
        n137 = Index Array(array=w349) -> (element=w353:waveform(dbl))  [unwired: 1 in]
        n138 = call <userlib>:"getAOwfm.vi"("error in (no error)"=w361, "Instrument.Lockin in"=w364) -> ("error out"=w359:errorcluster, "AO Waveforrm"=w346:waveform(dbl)[])  [unwired: 7 in, 1 out]
        n139 = Unbundle By Name(w353) -> ("Y"=w352:dbl[], "t0"=w354:timestamp, "dt"=w355:dbl)
        n140 = To Double Precision Float(number=w354) -> (double precision float=w356:dbl)
        n141 = for {
          tunnel: w355 -> [w385]
          tunnel: w356 -> [w383]
          tunnel: [w382] -> w348 mode=indexing
          tunnel: w352 -> [_] mode=indexing
          i -> [w386]
          n142 = Multiply(x=w386, y=w385) -> (x*y=w384:dbl)
          n143 = Add(x=w383, y=w384) -> (x+y=w382:dbl)
        }
        n144 = Bundle By Name(cluster=w351, "AI Waveform"=w349, "AOconfig"=w357, "AO Waveforrm"=w346, "time"=w348) -> (w350:T9)
        n145 = call <vilib>:"Add State(s) to Queue__jki_lib_state_machine.vi"("State(s) in (\"\")"=w366) -> ("States Out"=w365:string)  [unwired: 14 in]
      }
      frame "Measure: Filter and Decimate" {
        # "B"
        # "B"
        # "Template Separator\n(You can make a copy of, or modify, this frame)"
        n146 = Unbundle By Name(w390) -> ("time"=w395:dbl[], "AI Waveform"=w396:waveform(dbl)[])
        n147 = Unbundle By Name(w390) -> ("AO Waveforrm"=w394:waveform(dbl)[])
        n148 = for {
          tunnel: w396 -> [w419] mode=indexing
          tunnel: [w420] -> w399 mode=indexing
          tunnel: "offset" -> [w416] mode=indexing
          tunnel: "invert" -> [w418] mode=indexing
          n149 = Multiply(x=w419, y=w418) -> (x*y=w417:waveform(dbl))
          n150 = Add(x=w417, y=w416) -> (x+y=w420:waveform(dbl))
        }
        n151 = call "Decimate and Filter.vi"("Enabled?"="Enable Filter?", "low cutoff freq: fl"="low cutoff freq: fl", "decimating factor"="decimating factor", "Waveform in"=w395) -> ("Decimated and Filtered Array"=w393:dbl[])  [unwired: 6 in, 1 out]
        n152 = for {
          tunnel: "low cutoff freq: fl" -> [w405]
          tunnel: w394 -> [w409] mode=indexing
          tunnel: [w407] -> w391 mode=concatenating
          tunnel: "decimating factor" -> [w406]
          tunnel: "Enable Filter?" -> [w404]
          n153 = call "Decimate and Filter.vi"("Enabled?"=w404, "low cutoff freq: fl"=w405, "decimating factor"=w406, "Waveform in"=w409) -> ("Decimated and Filtered Array"=w408:dbl[])  [unwired: 6 in, 1 out]
          n154 = Build Cluster Array(w408) -> (w407:cluster{"Decimated and Filtered Array":dbl[]}[])
        }
        n155 = for {
          tunnel: "low cutoff freq: fl" -> [w411]
          tunnel: w399 -> [w415] mode=indexing
          tunnel: [w413] -> w392 mode=concatenating
          tunnel: "decimating factor" -> [w412]
          tunnel: "Enable Filter?" -> [w410]
          n156 = call "Decimate and Filter.vi"("Enabled?"=w410, "low cutoff freq: fl"=w411, "decimating factor"=w412, "Waveform in"=w415) -> ("Decimated and Filtered Array"=w414:dbl[])  [unwired: 6 in, 1 out]
          n157 = Build Cluster Array(w414) -> (w413:cluster{"Decimated and Filtered Array":dbl[]}[])
        }
        n158 = Bundle By Name(cluster=w390, "time (filtered)"=w393, "AI (filtered)"=w392, "AO (filtered)"=w391) -> (w389:T9)
        n159 = call <vilib>:"Add State(s) to Queue__jki_lib_state_machine.vi"("State(s) in (\"\")"=w403) -> ("States Out"=w402:string)  [unwired: 14 in]
      }
      frame "---------- File ----------" {
        # "Do not put any code in this frame.\n(It is a separator no-op. You can make a copy of this frame to create a new Macro frame)"
        n160 = call <vilib>:"Add State(s) to Queue__jki_lib_state_machine.vi"("State(s) in (\"\")"=w424) -> ("States Out"=w423:string)  [unwired: 14 in]
      }
      frame "File: Save" {
        w425 = FALSE  # append?
        # "Do not put any code in this frame.\n(It is a separator no-op. You can make a copy of this frame to create a new Macro frame)"
        n161 = Unbundle By Name(w438) -> ("Execution:State"=w426:T10, "Control Experiment"=w443:refnum<class "SMO.Control Experiment.lvclass">, "time (filtered)"=w436:dbl[], "AI (filtered)"=w429:cluster{"Decimated and Filtered Array":dbl[]}[], "AO (filtered)"=w431:cluster{"Decimated and Filtered Array":dbl[]}[])
        n162 = Array Size(array=w429) -> (size(s)=w428:i32)
        n163 = Array Size(array=w431) -> (size(s)=w430:i32)
        n164 = call "Create Keys (AI).vi"("Numeric"=w428) -> ("AI Keys"=w433:string[])  [unwired: 2 in]
        n165 = call "Create Keys (AO).vi"("Numeric"=w430) -> ("AO Keys"=w432:string[])  [unwired: 2 in]
        n166 = Build Cluster Array(w436) -> (w440:cluster{"time (filtered)":dbl[]}[])
        n167 = Build Array (concatenate)("time" ("wavenames"), w433, w432) -> (w434:string[])
        n168 = Build Array (concatenate)(w440, w429, w431) -> (w427:cluster{"Decimated and Filtered Array":dbl[]}[])
        n169 = for {
          tunnel: w434 -> [w451] mode=indexing
          tunnel: w427 -> [w450] mode=indexing
          tunnel: [w449] -> w441
          tunnel: w442 -> [w448]
          shift-right: [w452] -> w444
          shift-left: w443 -> [w453]
          n170 = call "Write Dictionary Element.vi"("error in (no error)"=w448, "value"=w450, "key"=w451, "Control Experiment"=w453) -> ("error out"=w449:errorcluster, "Control Experiment out"=w452:refnum<class "SMO.Control Experiment.lvclass">)  [unwired: 6 in]
        }
        n171 = call "Exec State to Append.vi"("Execution:State"=w426) -> ()  [unwired: 2 in, 1 out]
        n172 = call "Save Transport TDMS File.vi"("error in (no error)"=w441, "append?"=w425, "Control Experiment"=w444) -> ("error out"=w445:errorcluster, "Control Experiment out"=w439:refnum<class "SMO.Control Experiment.lvclass">)  [unwired: 7 in]
        n173 = Bundle By Name(cluster=w438, "Control Experiment"=w439) -> (w437:T9)
        n174 = call <vilib>:"Add State(s) to Queue__jki_lib_state_machine.vi"("State(s) in (\"\")"=w447) -> ("States Out"=w446:string)  [unwired: 14 in]
      }
    }
  }
  "error out" <- w1
  n175 = Unbundle By Name(w4) -> ("Transport"=→"Transport out":refnum<class "SMO.Transport.lvclass">)
